vi "A33ConfigurePulse.vi"(5 "Trailing edge":dbl=4e-09 format="%#_12g", 6 "Pulse width":dbl=0.1 format="%#_12g", 7 "Leading edge":dbl=4e-09 format="%#_12g", 8 "error in (no error)":errorcluster, 9 "Pulse period":dbl=1.0 format="%#_12g", 10 "Channel (1: Channel1)":u16(ring)=1 items=["Channel1"=1, "Channel2"=2], 11 "VISA resource name":refnum<visa-resource-name>) -> (0 "error out":errorcluster, 3 "VISA resource name out":refnum<visa-resource-name>)   [LabVIEW 2022 SP3]
doc: "Selects the waveform shape, frequency, amplitude, offset, and phase for a standard waveform."
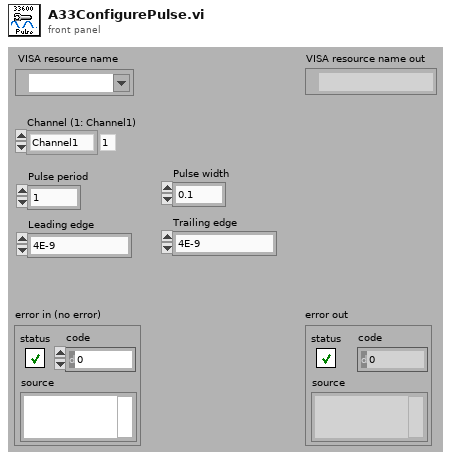
[diagram p1: front panel]
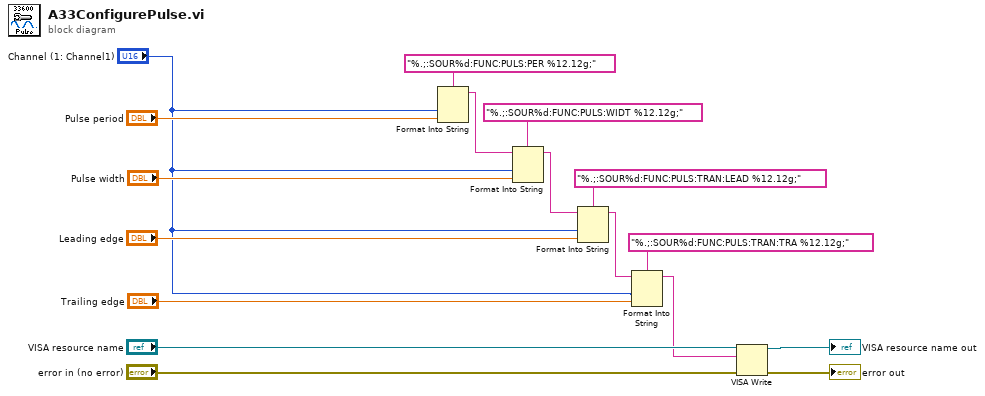
[diagram p0: block diagram]
diagram:
  n1 = Format Into String(format string="%.;:SOUR%d:FUNC:PULS:PER %12.12g;", "Channel (1: Channel1)", "Pulse period") -> (resulting string=w14:string)  [unwired: 2 in, 1 out]
  n2 = Format Into String(format string="%.;:SOUR%d:FUNC:PULS:WIDT %12.12g;", initial string=w14, "Channel (1: Channel1)", "Pulse width") -> (resulting string=w12:string)  [unwired: 1 in, 1 out]
  n3 = Format Into String(format string="%.;:SOUR%d:FUNC:PULS:TRAN:LEAD %12.12g;", initial string=w12, "Channel (1: Channel1)", "Leading edge") -> (resulting string=w2:string)  [unwired: 1 in, 1 out]
  n4 = Format Into String(format string="%.;:SOUR%d:FUNC:PULS:TRAN:TRA %12.12g;", initial string=w2, "Channel (1: Channel1)", "Trailing edge") -> (resulting string=w1:string)  [unwired: 1 in, 1 out]
  n5 = VISA Write(VISA resource name="VISA resource name", write buffer=w1, error in (no error)="error in (no error)") -> (VISA resource name out=→"VISA resource name out":refnum<visa-resource-name>, error out=→"error out":errorcluster)  [unwired: 1 out]
